vi "Read Logic Datas.vi"(8 "error in (no error)":errorcluster, 10 "length":u32, 11 "buffer":i8[](array[numeric])=array[1048576 elements]) -> (0 "error out":errorcluster, 2 "function return":u32, 3 "buffer out":i8[](array[numeric]))   [LabVIEW 2021, in "vmmso.lvlib"]
doc: "DLL_API unsigned int WINAPI ReadLogicDatas(unsigned char* buffer, unsigned int length);"
uses:
  vmmso.lvlib
  vmmso.dll
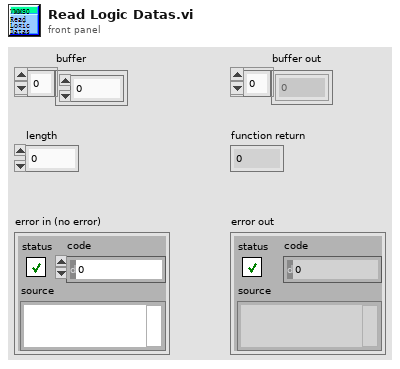
[diagram p1: front panel]
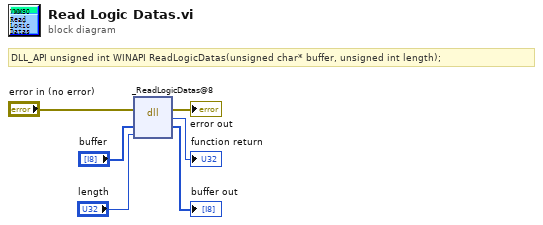
[diagram p0: block diagram]
diagram:
  # "DLL_API unsigned int WINAPI ReadLogicDatas(unsigned char* buffer, unsigned int length);"
  n1 = dll-call lib="O:/MSO/library/demo-Labview/vmmso/vmmso.*" fn="_ReadLogicDatas@8"(error in="error in (no error)", "buffer"="buffer", "length"="length") -> (error out=→"error out":errorcluster, →"function return":u32, "buffer"=→"buffer out":i8[])  [unwired: 3 in, 1 out]
